vi "Resize Array Indicator.vi"(10 "Max Rows (-1)":i32=-1, 11 "Arr Refnum":refnum<vi>) -> ()   [LabVIEW 2017]
doc: "This VI resizes an array indicator or control at runtime to the smaller of either Max Rows or Array Size. If the Array Size exceeds Max Rows the vi trims the indicator or control to Max Rows and enables the vertical scroll bar. If Max Rows is not supplied the default value is -1 and the array will resize to Array Size."
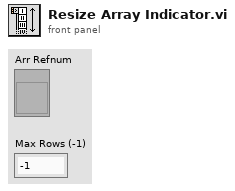
[diagram p1: front panel]
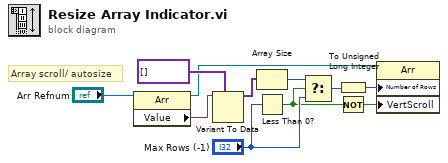
[diagram p0: block diagram]
diagram:
  # "Array scroll/ autosize"
  n1 = property class="Arr"(reference="Arr Refnum") -> (reference out=w8:refnum<vi>, "Value"=w11:variant)  [unwired: 1 in, 1 out]
  n2 = Variant To Data(type=variant[] [], Variant=w11) -> (data=w9:variant[])  [unwired: 1 in, 1 out]
  n3 = Array Size(array=w9) -> (size(s)=w7:i32)
  n4 = Less Than 0?(x="Max Rows (-1)") -> (x < 0?=w1:bool)
  n5 = Select(t=w7, s=w1, f="Max Rows (-1)") -> (s? t:f=w6:i32)
  n6 = To Unsigned Long Integer(number=w6) -> (unsigned 32bit integer=w4:u32)
  n7 = Not(x=w1) -> (.not. x?=w5:bool)
  n8 = property class="Arr"(reference=w8, "Number of Rows"=w4, "VertScroll"=w5) -> ()  [unwired: 1 in, 2 out]
